vi "DataRequest_from_Gviewer.vi"(7 "Periodic?":bool, 8 "error in (no error)":errorcluster, 9 "Sending Gviewer":string, 10 "DataRequest":T1, 11 "Gserver in":refnum<class "Gserver.lvclass">) -> (0 "error out":errorcluster, 3 "Gserver out":refnum<class "Gserver.lvclass">)   [LabVIEW 2020, in "Gserver.lvclass"]
doc: "Andre Koelewijn, 16 jan 2021\n\nProcess a query from one of the Gviewer instances.\nBased upon this query this VI must determine from which FAMM resolution layer data is needed.\nThe FAMM class will determine if the request can be fetched from RAM memory or if it must be retrieved from disk."
uses:
  Gserver.lvclass
  Gview/controls/Typedef_datarequest.ctl
  Gview/controls/Typedef_Live.ctl
  Gserver.lvclass/Gserver.ctl
  FAMM/controls/FAMMrequest.ctl
  FAMM/controls/typedef-functions.ctl
  controls/Typedef_PeriodicUpdate.ctl
  FAMM/FAMM.lvclass
  Gview/Gviewer.lvclass
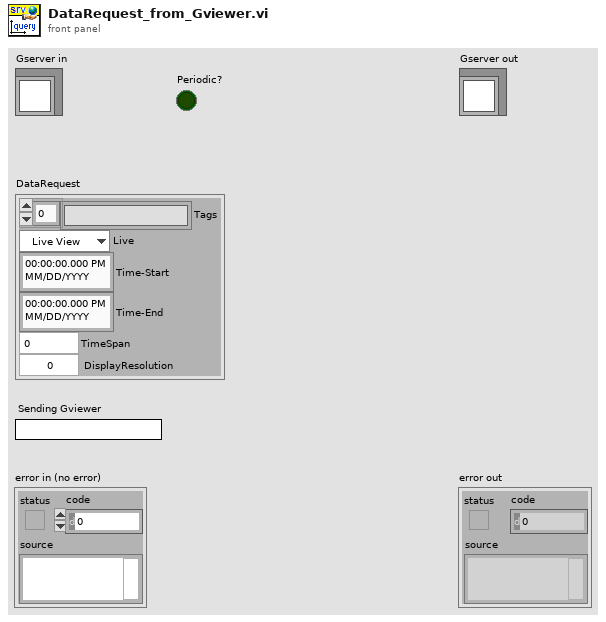
[diagram p1: front panel]
types:
  T1 = typedef "Gviewer.lvclass/Typedef_datarequest.ctl" = cluster{"Tags":string[], "Live":T2, "Time-Start":timestamp, "Time-End":timestamp, "TimeSpan":dbl, "DisplayResolution":i32}
  T2 = typedef "Gviewer.lvclass/Typedef_Live.ctl" = enum16{"Live View", "Freeze"}
  T3 = typedef "typedef-functions.ctl" = enum16{"PAQ-request", "PAQ-taglist-request", "WAQ-request", "EAQ-request", "TAG-based-request", "PAQ-MemoryMap", "Exit-FAMM"}
  T4 = typedef "FAMM.lvclass/FAMMrequest.ctl" = cluster{"Tags":string[], "Time-Start":timestamp, "Time-End":timestamp, "Live":T2, "TimeSpan":dbl, "DisplayResolution":i32}
  T5 = typedef "Gserver.lvclass/Typedef_PeriodicUpdate.ctl" = cluster{"Sending Gviewer":string, "PreviousUpdate":timestamp, "UpdateRate":dbl, "DataRequest":T1}
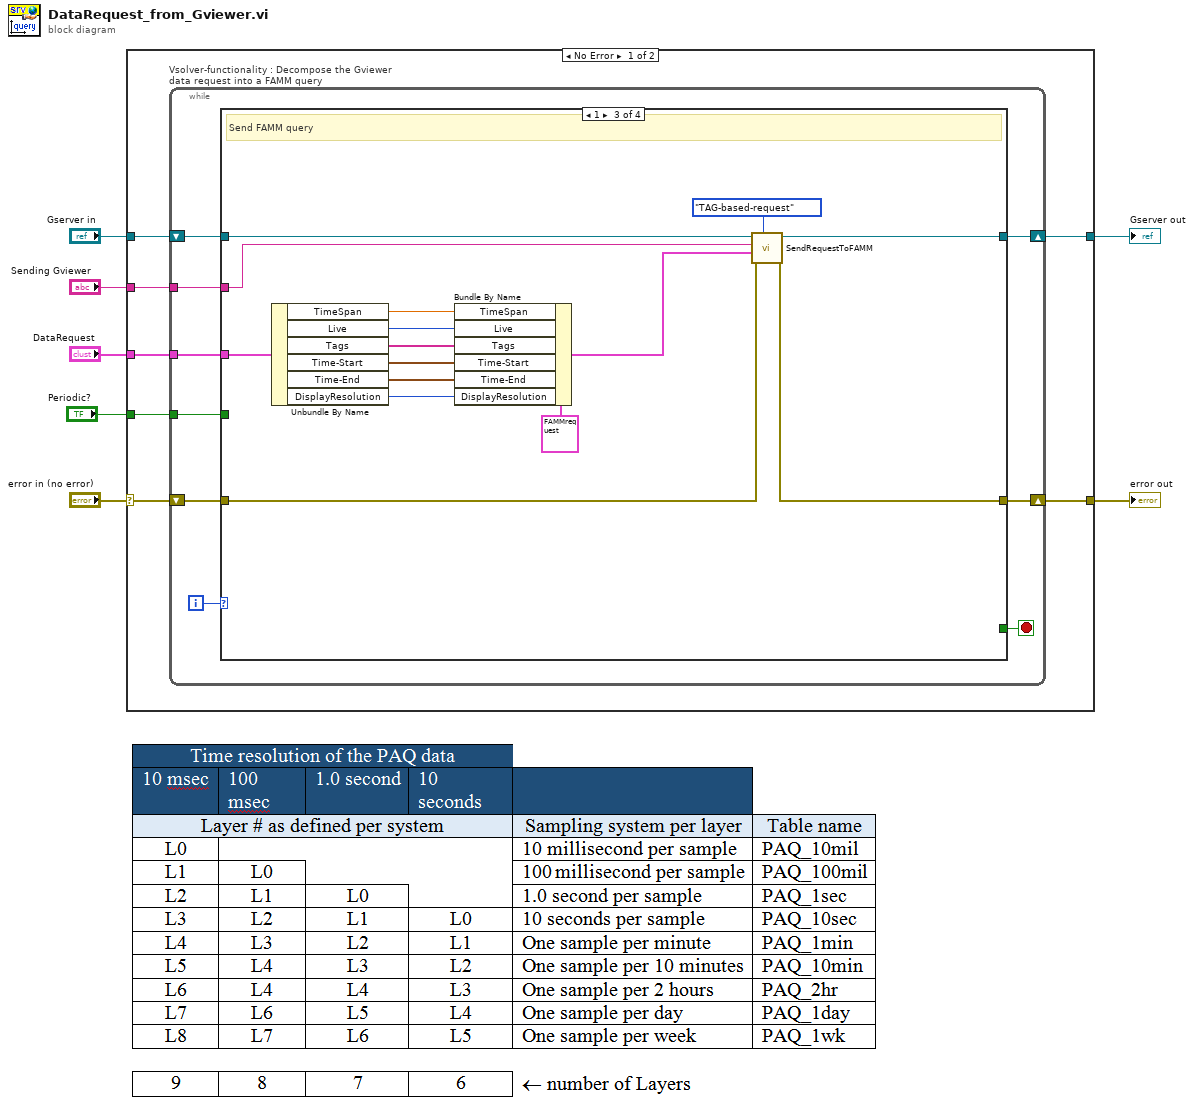
[diagram p0: block diagram]
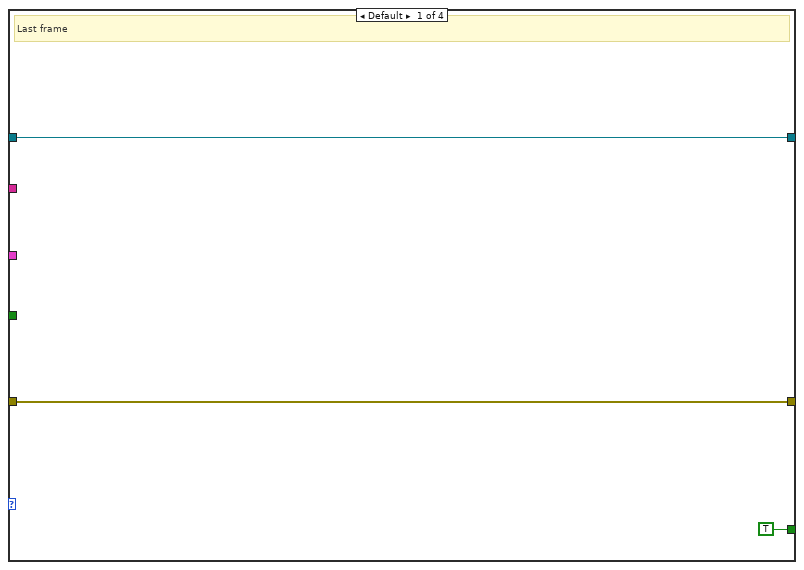
[diagram p2: hidden frame]
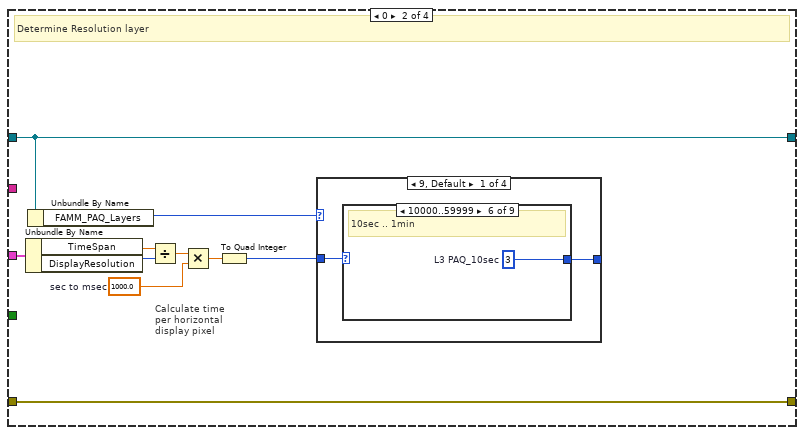
[diagram p3: hidden frame]
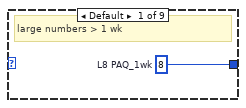
[diagram p4: hidden frame]
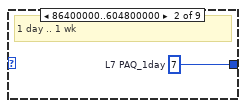
[diagram p5: hidden frame]
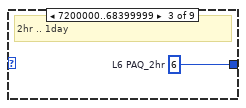
[diagram p6: hidden frame]
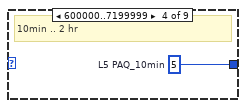
[diagram p7: hidden frame]
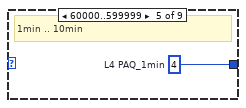
[diagram p8: hidden frame]
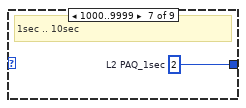
[diagram p9: hidden frame]
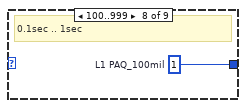
[diagram p10: hidden frame]
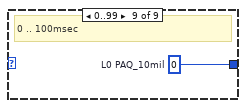
[diagram p11: hidden frame]
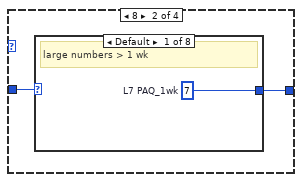
[diagram p12: hidden frame]
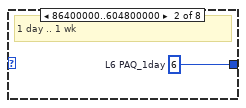
[diagram p13: hidden frame]
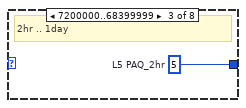
[diagram p14: hidden frame]
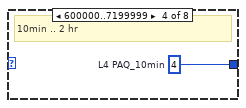
[diagram p15: hidden frame]
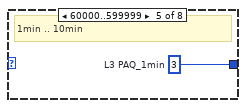
[diagram p16: hidden frame]
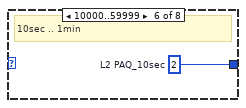
[diagram p17: hidden frame]
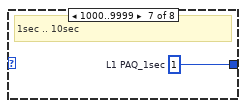
[diagram p18: hidden frame]
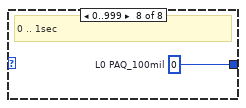
[diagram p19: hidden frame]
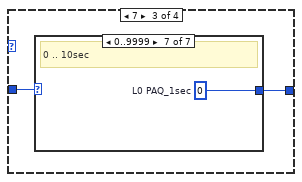
[diagram p20: hidden frame]
diagram:
  n1 = case shown="No Error" "error in (no error)" {
    selector: "error in (no error)" -> [w13 w154]
    tunnel: [w11 w154] -> w6
    tunnel: [w12 w153] -> w4
    tunnel: "Gserver in" -> [w14 w153]
    tunnel: "Sending Gviewer" -> [w9 _]
    tunnel: "DataRequest" -> [w10 _]
    tunnel: "Periodic?" -> [w8 _]
    frame No Error {
      n2 = while "Vsolver-functionality : Decompose the Gviewer data request into a FAMM query" {
        shift-right: [w19] -> w11
        shift-left: w13 -> [w21]
        shift-right: [w18] -> w12
        shift-left: w14 -> [w22]
        tunnel: w10 -> [w17]
        tunnel: w9 -> [w16]
        tunnel: w8 -> [w15]
        i -> [w23]
        stop <- w20 stop-if-true
        n3 = case shown="1" w23 {
          tunnel: w22 -> [w24 w30 w83 w96]
          tunnel: w21 -> [w25 w36 w78 w95]
          tunnel: [TRUE _ _ _] -> w20
          tunnel: [w25 w36 w79 w93] -> w19
          tunnel: [w24 w30 w84 w94] -> w18
          tunnel: w17 -> [_ w35 w88 w92]
          tunnel: w16 -> [_ _ w81 w91]
          tunnel: w15 -> [_ _ _ w90]
          frame Default {
            # "Last frame"
          }
          frame 0 {
            w31 = 1000.0  # sec to msec
            # "Calculate time\nper horizontal\ndisplay pixel"
            # "Determine Resolution layer"
            n4 = Unbundle By Name(w35) -> ("TimeSpan"=w34:dbl, "DisplayResolution"=w33:i32)
            n5 = Unbundle By Name(w30) -> ("FAMM_PAQ_Layers"=w29:i32)
            n6 = Divide(x=w34, y=w33) -> (x/y=w32:dbl)
            n7 = Multiply(x=w32, y=w31) -> (x*y=w28:dbl)
            n8 = To Quad Integer(1:w28) -> (0:w27:i64)
            n9 = case shown="9, Default" w29 {
              tunnel: w27 -> [w38 w49 w59 w68]
              tunnel: [w37 w48 w58 w67] -> _
              frame 9, Default {
                n10 = case shown="10000..59999" w38 {
                  tunnel: [w39 w40 w41 w42 w43 w44 w45 w46 w47] -> w37
                  frame Default {
                    w39 = 8  # L8 PAQ_1wk
                    # "large numbers > 1 wk"
                  }
                  frame 86400000..604800000 {
                    w40 = 7  # L7 PAQ_1day
                    # "1 day .. 1 wk"
                  }
                  frame 7200000..68399999 {
                    w41 = 6  # L6 PAQ_2hr
                    # "2hr .. 1day"
                  }
                  frame 600000..7199999 {
                    w42 = 5  # L5 PAQ_10min
                    # "10min .. 2 hr"
                  }
                  frame 60000..599999 {
                    w43 = 4  # L4 PAQ_1min
                    # "1min .. 10min"
                  }
                  frame 10000..59999 {
                    w44 = 3  # L3 PAQ_10sec
                    # "10sec .. 1min"
                  }
                  frame 1000..9999 {
                    w45 = 2  # L2 PAQ_1sec
                    # "1sec .. 10sec"
                  }
                  frame 100..999 {
                    w46 = 1  # L1 PAQ_100mil
                    # "0.1sec .. 1sec"
                  }
                  frame 0..99 {
                    w47 = 0  # L0 PAQ_10mil
                    # "0 .. 100msec"
                  }
                }
              }
              frame 8 {
                n11 = case shown="Default" w49 {
                  tunnel: [w50 w51 w52 w53 w54 w55 w56 w57] -> w48
                  frame Default {
                    w50 = 7  # L7 PAQ_1wk
                    # "large numbers > 1 wk"
                  }
                  frame 86400000..604800000 {
                    w51 = 6  # L6 PAQ_1day
                    # "1 day .. 1 wk"
                  }
                  frame 7200000..68399999 {
                    w52 = 5  # L5 PAQ_2hr
                    # "2hr .. 1day"
                  }
                  frame 600000..7199999 {
                    w53 = 4  # L4 PAQ_10min
                    # "10min .. 2 hr"
                  }
                  frame 60000..599999 {
                    w54 = 3  # L3 PAQ_1min
                    # "1min .. 10min"
                  }
                  frame 10000..59999 {
                    w55 = 2  # L2 PAQ_10sec
                    # "10sec .. 1min"
                  }
                  frame 1000..9999 {
                    w56 = 1  # L1 PAQ_1sec
                    # "1sec .. 10sec"
                  }
                  frame 0..999 {
                    w57 = 0  # L0 PAQ_100mil
                    # "0 .. 1sec"
                  }
                }
              }
              frame 7 {
                n12 = case shown="0..9999" w59 {
                  tunnel: [w60 w61 w62 w63 w64 w65 w66] -> w58
                  frame Default {
                    w60 = 6  # L6 PAQ_1wk
                    # "large numbers > 1 wk"
                  }
                  frame 86400000..604800000 {
                    w61 = 5  # L5PAQ_1day
                    # "1 day .. 1 wk"
                  }
                  frame 7200000..68399999 {
                    w62 = 4  # L4 PAQ_2hr
                    # "2hr .. 1day"
                  }
                  frame 600000..7199999 {
                    w63 = 3  # L3 PAQ_10min
                    # "10min .. 2 hr"
                  }
                  frame 60000..599999 {
                    w64 = 2  # L2 PAQ_1min
                    # "1min .. 10min"
                  }
                  frame 10000..59999 {
                    w65 = 1  # L1 PAQ_10sec
                    # "10sec .. 1min"
                  }
                  frame 0..9999 {
                    w66 = 0  # L0 PAQ_1sec
                    # "0 .. 10sec"
                  }
                }
              }
              frame 6 {
                n13 = case shown="Default" w68 {
                  tunnel: [w69 w70 w71 w72 w73 w74] -> w67
                  frame Default {
                    w69 = 5  # L5 PAQ_1wk
                    # "large numbers > 1 wk"
                  }
                  frame 86400000..604800000 {
                    w70 = 4  # L4PAQ_1day
                    # "1 day .. 1 wk"
                  }
                  frame 7200000..68399999 {
                    w71 = 3  # L3 PAQ_2hr
                    # "2hr .. 1day"
                  }
                  frame 600000..7199999 {
                    w72 = 2  # L2 PAQ_10min
                    # "10min .. 2 hr"
                  }
                  frame 60000..599999 {
                    w73 = 1  # L1 PAQ_1min
                    # "1min .. 10min"
                  }
                  frame 0..59999 {
                    w74 = 0  # L0 PAQ_10sec
                    # "10sec .. 1min"
                  }
                }
              }
            }
          }
          frame 1 {
            # "Send FAMM query"
            n14 = Unbundle By Name(w88) -> ("TimeSpan"=w76:dbl, "Live"=w77:T2, "Tags"=w87:string[], "Time-Start"=w86:timestamp, "Time-End"=w85:timestamp, "DisplayResolution"=w75:i32)
            n15 = Bundle By Name(cluster=T4 {"Tags"=["ch0001", "ch0002", "ch0003", "ch0004", "ch0005"], "Time-Start"=timestamp(3693712856.876272 s since 1904-01-01), "Time-End"=timestamp(3693716456.876272 s since 1904-01-01), "Live"=enum."Live View", "TimeSpan"=0.0, "DisplayResolution"=0} ("PAQ-request"), "TimeSpan"=w76, "Live"=w77, "Tags"=w87, "Time-Start"=w86, "Time-End"=w85, "DisplayResolution"=w75) -> (w80:T4)
            n16 = call "SendRequestToFAMM.vi"("FAMM-function"=typedef-functions."TAG-based-request", "error in (no error)"=w78, "Data"=w80, "Source"=w81, "Gserver in"=w83) -> ("error out"=w79:errorcluster, "Gserver out"=w84:refnum<class "Gserver.lvclass">)  [unwired: 5 in]
          }
          frame 2 {
            # "update live updates"
            n17 = case shown="False" w90 {
              tunnel: w96 -> [w105 w152]
              tunnel: w95 -> [w104 w151]
              tunnel: [w100 w152] -> w94
              tunnel: [w99 w151] -> w93
              tunnel: w92 -> [w98 _]
              tunnel: w91 -> [w97 _]
              frame False {
                n18 = call "CheckLiveUpdates.vi"("error in (no error)"=w104, "GraphName"=w97, "Gserver in"=w105) -> ("error out"=w101:errorcluster, "index"=w103:i32, "Gserver out"=w102:refnum<class "Gserver.lvclass">)  [unwired: 6 in]
                n19 = Unbundle By Name(w98) -> ("Live"=w106:T2)
                n20 = case shown="\"Freeze\"" w106 {
                  tunnel: w103 -> [w113 w141]
                  tunnel: w102 -> [w112 w140]
                  tunnel: w101 -> [w110 w139]
                  tunnel: [w111 w138] -> w100
                  tunnel: [w109 w137] -> w99
                  tunnel: w98 -> [w108 _]
                  tunnel: w97 -> [w107 _]
                  frame "Live View" {
                    n21 = case shown="Default" w113 {
                      selector: w113 -> [w123 _]
                      tunnel: w112 -> [w120 w132]
                      tunnel: [w121 w133] -> w111
                      tunnel: w110 -> [w125 w136]
                      tunnel: [w125 w136] -> w109
                      tunnel: w108 -> [w115 w127]
                      tunnel: w107 -> [w118 w129]
                      frame Default {
                        n22 = Get Date/Time In Seconds() -> (seconds since 1Jan1904=w117:timestamp)
                        n23 = Unbundle By Name(w120) -> ("PeriodicUpdates"=w124:T5[])
                        n24 = Bundle By Name(cluster=T5 {"Sending Gviewer"="", "PreviousUpdate"=timestamp(0 s since 1904-01-01), "UpdateRate"=0.0, "DataRequest"={"Tags"=[], "Live"=enum."Live View", "Time-Start"=timestamp(0 s since 1904-01-01), "Time-End"=timestamp(0 s since 1904-01-01), "TimeSpan"=0.0, "DisplayResolution"=0}} ("PeriodicUPdate"), "Sending Gviewer"=w118, "DataRequest"=w115, "UpdateRate"=0.1, "PreviousUpdate"=w117) -> (w114:T5)
                        n25 = Replace Array Subset(array=w124, new element=w114, index=w123) -> (w122:T5[])
                        n26 = Bundle By Name(cluster=w120, "PeriodicUpdates"=w122) -> (w121:refnum<class "Gserver.lvclass">)
                      }
                      frame -1 {
                        n27 = Get Date/Time In Seconds() -> (seconds since 1Jan1904=w126:timestamp)
                        n28 = Unbundle By Name(w132) -> ("PeriodicUpdates"=w135:T5[])
                        n29 = Bundle By Name(cluster=T5 {"Sending Gviewer"="", "PreviousUpdate"=timestamp(0 s since 1904-01-01), "UpdateRate"=0.0, "DataRequest"={"Tags"=[], "Live"=enum."Live View", "Time-Start"=timestamp(0 s since 1904-01-01), "Time-End"=timestamp(0 s since 1904-01-01), "TimeSpan"=0.0, "DisplayResolution"=0}} ("PeriodicUPdate"), "Sending Gviewer"=w129, "DataRequest"=w127, "UpdateRate"=0.1, "PreviousUpdate"=w126) -> (w130:T5)
                        n30 = Build Array (concatenate)(w135, w130) -> (w134:T5[])
                        n31 = Bundle By Name(cluster=w132, "PeriodicUpdates"=w134) -> (w133:refnum<class "Gserver.lvclass">)
                      }
                    }
                  }
                  frame "Freeze" {
                    n32 = case shown="Default" w141 {
                      selector: w141 -> [w146 _]
                      tunnel: w140 -> [w142 w150]
                      tunnel: w139 -> [w148 w149]
                      tunnel: [w143 w150] -> w138
                      tunnel: [w148 w149] -> w137
                      frame Default {
                        n33 = Unbundle By Name(w142) -> ("PeriodicUpdates"=w147:T5[])
                        n34 = Delete From Array(array=w147, length=1, index=w146) -> (array with subset deleted=w144:T5[])  [unwired: 1 out]
                        n35 = Bundle By Name(cluster=w142, "PeriodicUpdates"=w144) -> (w143:refnum<class "Gserver.lvclass">)
                      }
                      frame -1 {
                      }
                    }
                  }
                }
              }
              frame True {
              }
            }
          }
        }
      }
    }
    frame Error {
    }
  }
  "error out" <- w6
  "Gserver out" <- w4
